vi "InitGUI.vi"(8 "error in (no error)":errorcluster, 10 "App Configuration":T1, 11 "GUI Refs":T2) -> (0 "error out":errorcluster)   [LabVIEW 2019]
uses:
  Typedefs/#cluster_GUIRefs.ctl
  Application Configuration VIs/#cluster_AppConfiguration.ctl
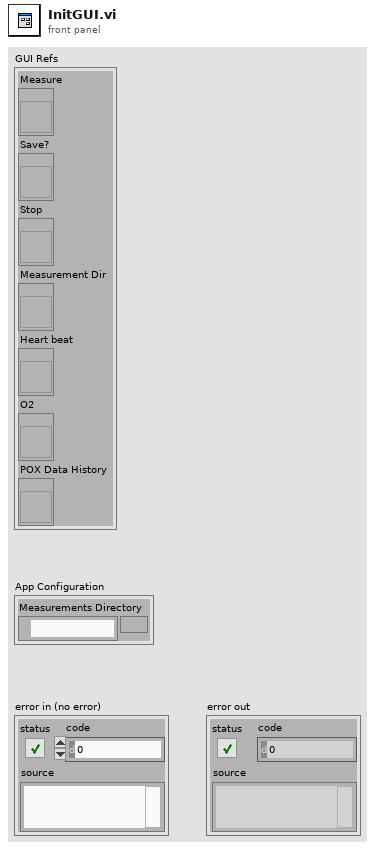
[diagram p1: front panel]
types:
  T1 = typedef "#cluster_AppConfiguration.ctl" = cluster{"Measurements Directory":path}
  T2 = typedef "#cluster_GUIRefs.ctl" = cluster{"Measure":refnum<vi>, "Save?":refnum<vi>, "Stop":refnum<vi>, "Measurement Dir":refnum<vi>, "Heart beat":refnum<vi>, "O2":refnum<vi>, "POX Data History":refnum<vi>}
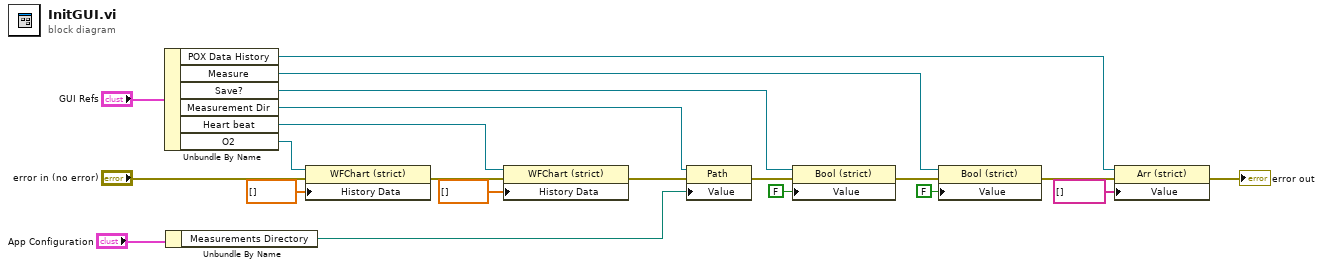
[diagram p0: block diagram]
diagram:
  n1 = Unbundle By Name("GUI Refs") -> ("POX Data History"=w5:refnum<vi>, "Measure"=w17:refnum<vi>, "Save?"=w16:refnum<vi>, "Measurement Dir"=w14:refnum<vi>, "Heart beat"=w11:refnum<vi>, "O2"=w7:refnum<vi>)
  n2 = Unbundle By Name("App Configuration") -> ("Measurements Directory"=w1:path)
  n3 = property class="WFChart (strict)"(reference=w7, error in="error in (no error)", "History Data"=dbl[] []) -> (error out=w10:errorcluster)  [unwired: 1 out]
  n4 = property class="WFChart (strict)"(reference=w11, error in=w10, "History Data"=dbl[] []) -> (error out=w13:errorcluster)  [unwired: 1 out]
  n5 = property class="Path"(reference=w14, error in=w13, "Value"=w1) -> (error out=w15:errorcluster)  [unwired: 1 out]
  n6 = property class="Bool (strict)"(reference=w16, error in=w15, "Value"=FALSE) -> (error out=w18:errorcluster)  [unwired: 1 out]
  n7 = property class="Bool (strict)"(reference=w17, error in=w18, "Value"=FALSE) -> (error out=w6:errorcluster)  [unwired: 1 out]
  n8 = property class="Arr (strict)"(reference=w5, error in=w6, "Value"=string[] []) -> (error out=→"error out":errorcluster)  [unwired: 1 out]
